vi "Initialize XML from File.vi"(8 "error in (no error)":errorcluster, 11 "XML File Path":path) -> (0 "error out":errorcluster, 3 "DOM document out":refnum<k20>)   [LabVIEW 2016, in "SLL File IO.lvlib"]
doc: "Initialize XML reference from a file path."
uses:
  SLL File IO.lvlib
  <vilib>/xml/NI_XML.lvlib
  <resource>/objmgr/DOMUserDefRef.rc
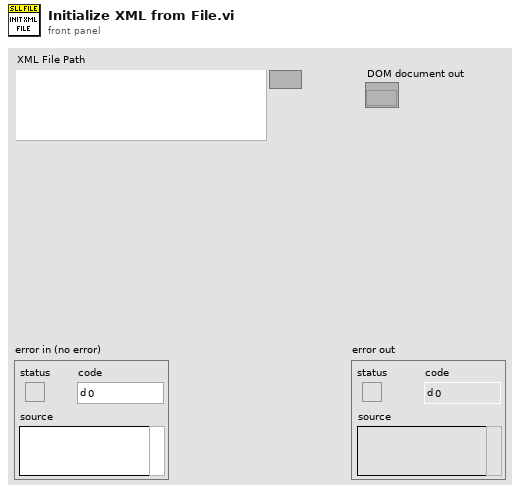
[diagram p1: front panel]
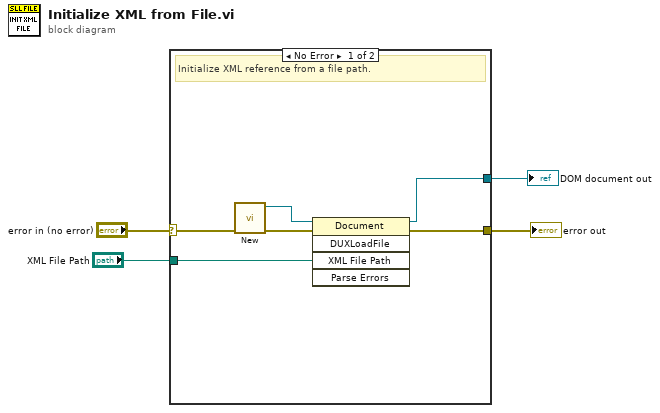
[diagram p0: block diagram]
diagram:
  n1 = case shown="No Error" "error in (no error)" {
    selector: "error in (no error)" -> [w10 w11]
    tunnel: [w8 w11] -> w3
    tunnel: "XML File Path" -> [w6 _]
    tunnel: [w5 _] -> w1
    frame No Error {
      # "Initialize XML reference from a file path."
      n2 = call <vilib>:"New.vi"("error in (no error)"=w10) -> ("error out"=w9:errorcluster, "DOM document out"=w7:refnum<k20>)  [unwired: 7 in]
      n3 = invoke class="Document" method="DUXLoadFile"(reference=w7, error in=w9, "XML File Path"=w6) -> (reference out=w5:refnum<k20>, error out=w8:errorcluster)  [unwired: 2 in, 3 out]
    }
    frame Error {
    }
  }
  "error out" <- w3
  "DOM document out" <- w1
